vi "Hardware-EPTx-Host.vi"() -> ()   [LabVIEW 2016]
uses:
  <vilib>/Powertrain Controls/Device Drivers/DCM/Rev0/FPGA/Digital Channel.ctl
  <vilib>/Powertrain Controls/Device Drivers/DCM/Rev0/FPGA/DCM - FPGA.lvlib
panel:
  in  "_EPTx Config List":i32(listbox) caption="Deployed EPTx Configurations"
  in  "_Refresh  EPTx Config":bool
  in  "_Open EPTx DB Editor":bool
  out "LoadingSettings":bool
  in  "LoadSettings":bool
  in  "_EPTx Signal Select":T2 caption="EPTx Signal Select"
  in  "HistoryCAD":u8=255
  in  "_Hidden":enum32{"Invisible"}(tab)
  in  "Aux4Select":u8
  in  "Aux3Select":u8
  in  "Aux2Select":u8
  in  "Aux1Select":u8
  in  "PrimarySelect":u8
  out "MaxCAD":sgl
  in  "SimSpeed":sgl
  in  "SimEnable":bool
  in  "SyncEnable":bool
  in  "ClearErrors":bool
  in  "Aux4Filter":sgl format="%#_6p"
  in  "Aux3Filter":sgl format="%#_6p"
  in  "Aux2Filter":sgl format="%#_6p"
  in  "Aux1Filter":sgl format="%#_6p"
  in  "PrimaryFilter":sgl format="%#_6p"
  out "RcvgPrimary":bool
  out "AuxWarning":bool
  out "WatchdogError":bool
  out "Config":bool
  out "PatternError":bool
  out "RatioError":bool
  out "Overflow":bool
  out "Stall":bool
  out "CurrentCAD":sgl
  out "Speed":sgl
  out "Sync":bool
  in  "EPTxSettingsFilename":string="c:\\ni-rt\\LabVIEW Data\\60-2.EPTx"
  out "SYS|Exec|IP_Address":string="10.15.1.12"
  in  "SYS|Exec|Password":string caption="Password"
  in  "SYS|Exec|Username":string="admin" caption="Username"
  in  "_EPTxState":T3 caption="EPTxState"
  out "_EPTx Data":T4 caption="EPTx Data"
  in  "_EPTxFilters":T5 caption="EPTxFilters" {"Aux 4 [s]" format="%#_6p"; "Aux 3 [s]" format="%#_6p"; "Aux 2 [s]" format="%#_6p"; "Aux 1 [s]" format="%#_6p"; "Primary [s]" format="%#_6p"}
  in  "StallSpeed":sgl=500.0
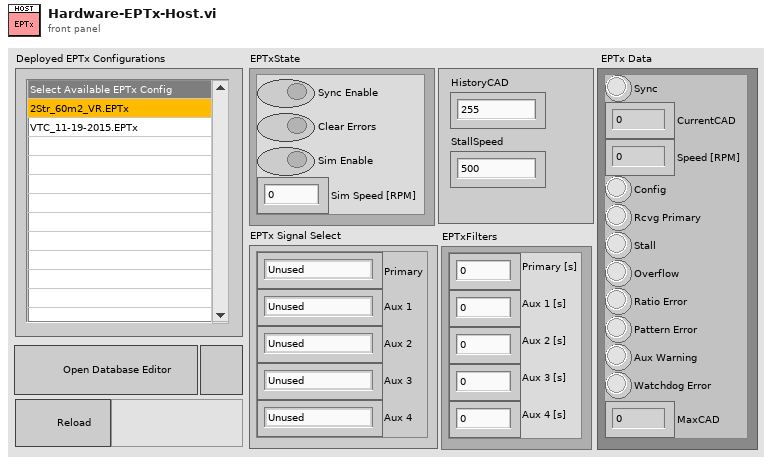
[diagram p1: front panel]
types:
  T1 = typedef "DCM - FPGA.lvlib/Digital Channel.ctl" = enum8{"Unused", "User OS", "Diff IO 1", "Diff IO 2", "Diff IO 3", "Diff IO 4", "Diff IO 5", "Diff IO 6", "Diff IO 7", "Diff IO 8", "Aux 1", "Aux 2", "Aux 3", "Aux 4", "Aux 5", "Aux 6", "Aux 7", "Aux 8", "Aux 9", "Aux 10", "Aux 11", "Aux 12", "Aux 13", "Aux 14", "Aux 15", "Aux 16"}
  T2 = cluster{"Primary":T1, "Aux 1":T1, "Aux 2":T1, "Aux 3":T1, "Aux 4":T1}
  T3 = cluster{"Sync Enable":bool, "Clear Errors":bool, "Sim Enable":bool, "Sim Speed [RPM]":sgl}
  T4 = cluster{"Sync":bool, "CurrentCAD":sgl, "Speed [RPM]":sgl, "Config":bool, "Rcvg Primary":bool, "Stall":bool, "Overflow":bool, "Ratio Error":bool, "Pattern Error":bool, "Aux Warning":bool, "Watchdog Error":bool, "MaxCAD":sgl}
  T5 = cluster{"Primary [s]":sgl, "Aux 1 [s]":sgl, "Aux 2 [s]":sgl, "Aux 3 [s]":sgl, "Aux 4 [s]":sgl}
  T6 = cluster{"PrimarySelect":u8, "Aux1Select":u8, "Aux2Select":u8, "Aux3Select":u8, "Aux4Select":u8}
  T7 = cluster{"PrimaryFilter":sgl, "Aux1Filter":sgl, "Aux2Filter":sgl, "Aux3Filter":sgl, "Aux4Filter":sgl}
  T8 = cluster{"Sync":bool, "CurrentCAD":sgl, "Speed":sgl, "Config":bool, "RcvgPrimary":bool, "Stall":bool, "Overflow":bool, "PatternError":bool, "RatioError":bool, "AuxWarning":bool, "WatchdogError":bool, "MaxCAD":sgl}
  T9 = cluster{"SyncEnable":bool, "ClearErrors":bool, "SimEnable":bool, "SimSpeed":sgl}
  T10 = typedef "LVMinMaxIncTypeDef.ctl" = cluster{"Minimum":dbl, "Maximum":dbl, "Increment":dbl}
  T11 = typedef "LVOutOfRangeActionTypeDef.ctl" = cluster{"OutOfRngActMin":u8, "OutOfRngActMax":u8, "OutOfRngActInc":u8}
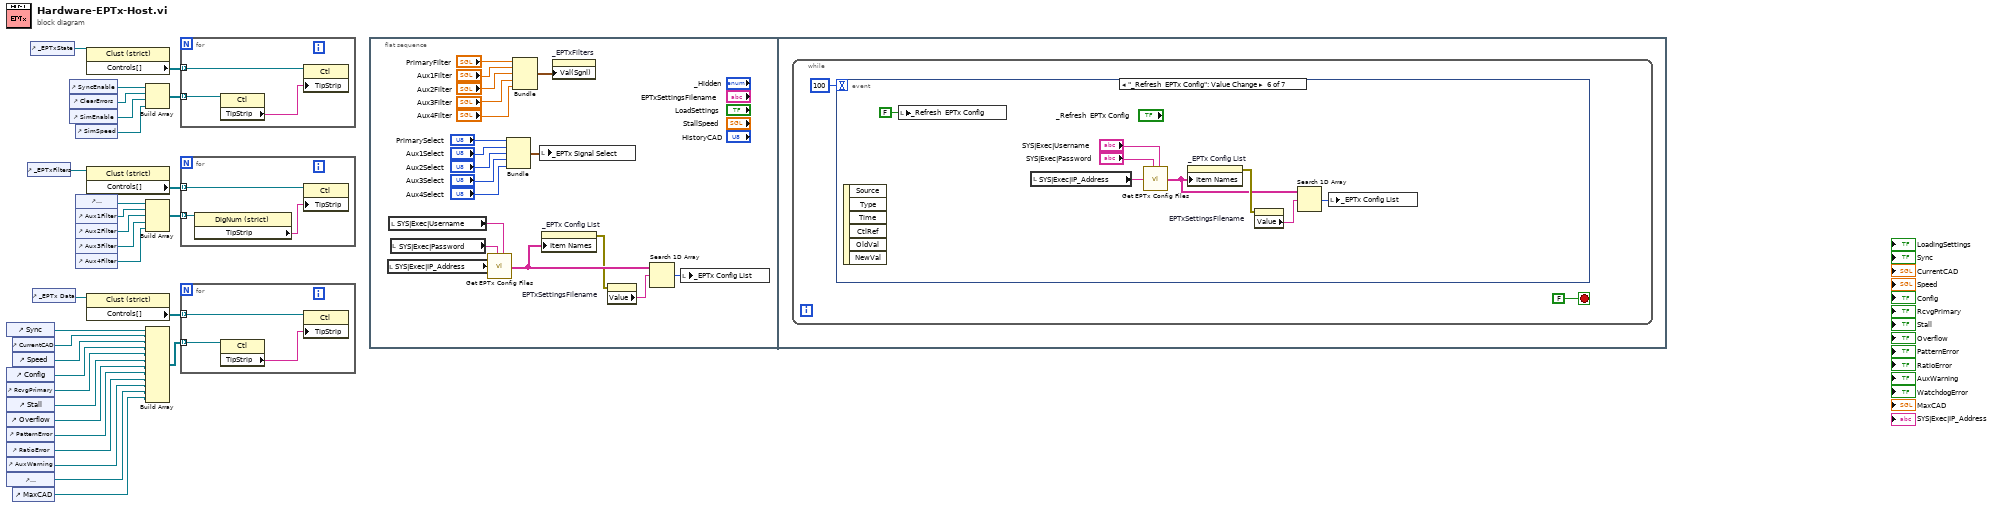
[diagram p0: block diagram]
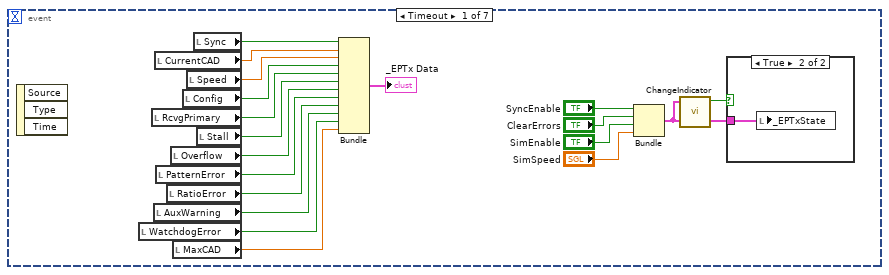
[diagram p2: hidden frame]
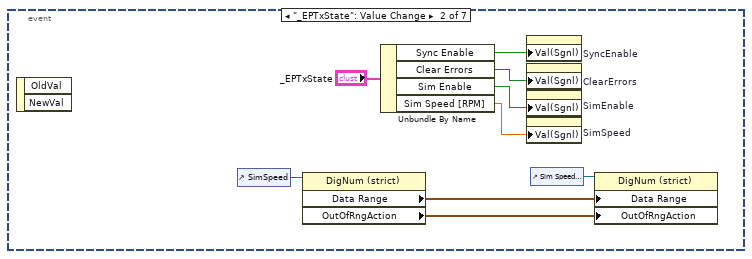
[diagram p4: hidden frame]
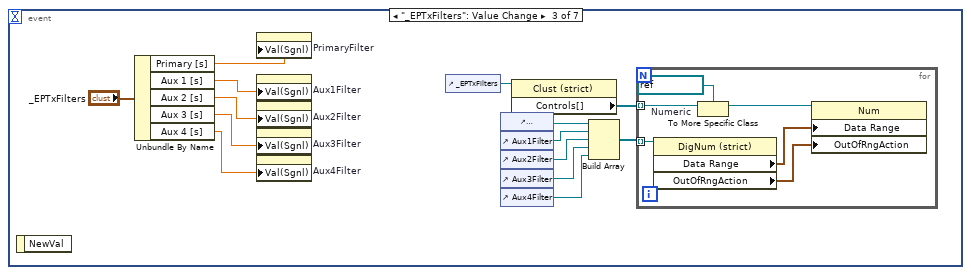
[diagram p5: hidden frame]
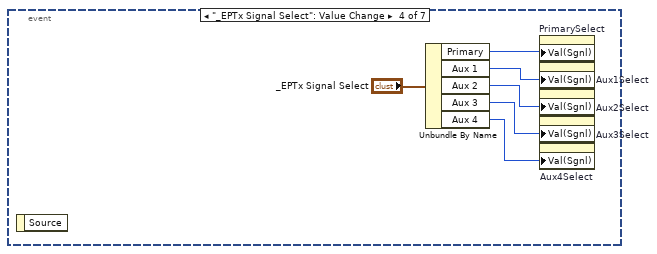
[diagram p6: hidden frame]
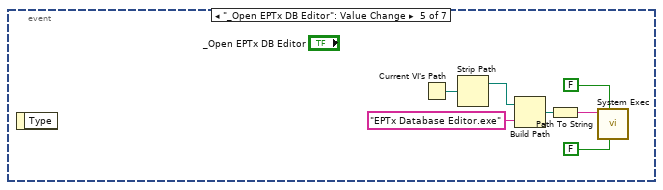
[diagram p7: hidden frame]
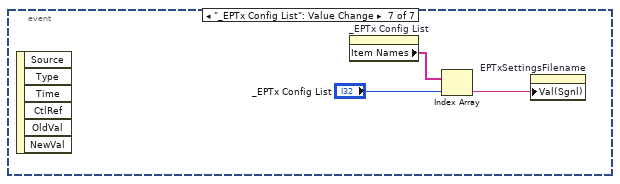
[diagram p8: hidden frame]
diagram:
  n1 = control-ref of="Sync"() -> (w12:refnum<vi>)
  n2 = control-ref of="Config"() -> (w9:refnum<vi>)
  n3 = control-ref of="RcvgPrimary"() -> (w8:refnum<vi>)
  n4 = control-ref of="Stall"() -> (w7:refnum<vi>)
  n5 = control-ref of="Overflow"() -> (w6:refnum<vi>)
  n6 = control-ref of="PatternError"() -> (w5:refnum<vi>)
  n7 = control-ref of="RatioError"() -> (w4:refnum<vi>)
  n8 = control-ref of="AuxWarning"() -> (w3:refnum<vi>)
  n9 = control-ref of="WatchdogError"() -> (w2:refnum<vi>)
  n10 = control-ref of="CurrentCAD"() -> (w11:refnum<vi>)
  n11 = control-ref of="Speed"() -> (w10:refnum<vi>)
  n12 = control-ref of="MaxCAD"() -> (w1:refnum<vi>)
  n13 = control-ref of="_EPTxFilters"() -> (w21:refnum<vi>)
  n14 = control-ref of="_EPTxState"() -> (w28:refnum<vi>)
  n15 = control-ref of="_EPTx Data"() -> (w13:refnum<vi>)
  n16 = control-ref of="SyncEnable"() -> (w27:refnum<vi>)
  n17 = control-ref of="ClearErrors"() -> (w26:refnum<vi>)
  n18 = control-ref of="SimEnable"() -> (w25:refnum<vi>)
  n19 = control-ref of="SimSpeed"() -> (w24:refnum<vi>)
  n20 = control-ref of="PrimaryFilter"() -> (w20:refnum<vi>)
  n21 = control-ref of="Aux1Filter"() -> (w19:refnum<vi>)
  n22 = control-ref of="Aux2Filter"() -> (w18:refnum<vi>)
  n23 = control-ref of="Aux3Filter"() -> (w17:refnum<vi>)
  n24 = control-ref of="Aux4Filter"() -> (w16:refnum<vi>)
  n25 = property on="Property Node" class="Clust (strict)"(reference=w28) -> ("Controls[]"=w30:refnum<vi>[])  [unwired: 1 in, 2 out]
  n26 = property on="Property Node" class="Clust (strict)"(reference=w21) -> ("Controls[]"=w22:refnum<vi>[])  [unwired: 1 in, 2 out]
  n27 = property on="Property Node" class="Clust (strict)"(reference=w13) -> ("Controls[]"=w15:refnum<vi>[])  [unwired: 1 in, 2 out]
  n28 = Build Array(w27, w26, w25, w24) -> (w29:refnum<vi>[])
  n29 = Build Array(w20, w19, w18, w17, w16) -> (w23:refnum<vi>[])
  n30 = Build Array(w12, w11, w10, w9, w8, w7, w6, w5, w4, w3, w2, w1) -> (w14:refnum<vi>[])
  n31 = for {
    tunnel: w30 -> [w33] mode=indexing
    tunnel: w29 -> [w31] mode=indexing
    n32 = property on="Property Node" class="Ctl"(reference=w31) -> ("TipStrip"=w32:string)  [unwired: 1 in, 2 out]
    n33 = property on="Property Node" class="Ctl"(reference=w33, "TipStrip"=w32) -> ()  [unwired: 1 in, 2 out]
  }
  n34 = for {
    tunnel: w22 -> [w36] mode=indexing
    tunnel: w23 -> [w34] mode=indexing
    n35 = property on="Property Node" class="DigNum (strict)"(reference=w34) -> ("TipStrip"=w35:string)  [unwired: 1 in, 2 out]
    n36 = property on="Property Node" class="Ctl"(reference=w36, "TipStrip"=w35) -> ()  [unwired: 1 in, 2 out]
  }
  n37 = for {
    tunnel: w15 -> [w39] mode=indexing
    tunnel: w14 -> [w37] mode=indexing
    n38 = property on="Property Node" class="Ctl"(reference=w37) -> ("TipStrip"=w38:string)  [unwired: 1 in, 2 out]
    n39 = property on="Property Node" class="Ctl"(reference=w39, "TipStrip"=w38) -> ()  [unwired: 1 in, 2 out]
  }
  n40 = flat-sequence {
    frame #0 {
      n41 = local read "SYS|Exec|IP_Address"() -> (w58:string)
      n42 = local read "SYS|Exec|Username"() -> (w56:string)
      n43 = local read "SYS|Exec|Password"() -> (w57:string)
      n44 = call "Get EPTx Config Files.vi"("password"=w57, "IP_Address"=w58, "username"=w56) -> ("EPTx Files"=w53:string[])  [unwired: 6 in]
      n45 = Bundle("PrimarySelect"="PrimarySelect", "Aux1Select"="Aux1Select", "Aux2Select"="Aux2Select", "Aux3Select"="Aux3Select", "Aux4Select"="Aux4Select") -> (w51:T6)  [unwired: 1 in]
      n46 = Bundle("PrimaryFilter"="PrimaryFilter", "Aux1Filter"="Aux1Filter", "Aux2Filter"="Aux2Filter", "Aux3Filter"="Aux3Filter", "Aux4Filter"="Aux4Filter") -> (w45:T7)  [unwired: 1 in]
      n47 = local write "_EPTx Signal Select"(w51) -> ()
      n48 = property on="_EPTx Config List" class="LstBox (strict)"("Item Names"=w53) -> (error out=w52:errorcluster)  [unwired: 2 in, 1 out]
      n49 = property on="_EPTxFilters" class="Clust (strict)"("Val(Sgnl)"=w45) -> ()  [unwired: 2 in, 2 out]
      n50 = property on="EPTxSettingsFilename" class="Str"(error in=w52) -> ("Value"=w55:string)  [unwired: 1 in, 2 out]
      n51 = Search 1D Array(1D array=w53, element=w55) -> (index of element=w54:i32)  [unwired: 1 in]
      n52 = local write "_EPTx Config List"(w54) -> ()
    }
    frame #1 {
      n53 = while {
        stop <- FALSE stop-if-true
        n54 = event shown="[5] \"_Refresh  EPTx Config\": Value Change" {
          selector: _ -> [_ _ _ _ _ _ _]
          dyn-events: _ -> [_ _ _ _ _ _ _]
          timeout: 100 -> [_ _ _ _ _ _ _]
          event Timeout {
            n55 = event-data() -> ()  [unwired: 1 in, 3 out]
            n56 = local read "WatchdogError"() -> (w79:bool)
            n57 = local read "RcvgPrimary"() -> (w73:bool)
            n58 = local read "AuxWarning"() -> (w78:bool)
            n59 = local read "CurrentCAD"() -> (w70:sgl)
            n60 = local read "PatternError"() -> (w76:bool)
            n61 = local read "RatioError"() -> (w77:bool)
            n62 = local read "Overflow"() -> (w75:bool)
            n63 = local read "MaxCAD"() -> (w68:sgl)
            n64 = local read "Config"() -> (w72:bool)
            n65 = local read "Speed"() -> (w71:sgl)
            n66 = local read "Sync"() -> (w69:bool)
            n67 = local read "Stall"() -> (w74:bool)
            n68 = Bundle("Sync"=w69, "CurrentCAD"=w70, "Speed"=w71, "Config"=w72, "RcvgPrimary"=w73, "Stall"=w74, "Overflow"=w75, "PatternError"=w76, "RatioError"=w77, "AuxWarning"=w78, "WatchdogError"=w79, "MaxCAD"=w68) -> (→"_EPTx Data":T8)  [unwired: 1 in]
            n69 = Bundle("SyncEnable"="SyncEnable", "ClearErrors"="ClearErrors", "SimEnable"="SimEnable", "SimSpeed"="SimSpeed") -> (w62:T9)  [unwired: 1 in]
            n70 = call "ChangeIndicator.vi"("Input"=w62) -> ("Change"=w61:bool)  [unwired: 9 in]
            n71 = case shown="True" w61 {
              tunnel: w62 -> [_ w80]
              frame False {
              }
              frame True {
                n72 = local write "_EPTxState"(w80) -> ()
              }
            }
          }
          event "_EPTxState": Value Change {
            n73 = event-data() -> ()  [unwired: 1 in, 2 out]
            n74 = control-ref of="SimSpeed"() -> (w84:refnum<vi>)
            n75 = property on="Property Node" class="DigNum (strict)"(reference=w84) -> ("Data Range"=w82:T10, "OutOfRngAction"=w81:T11)  [unwired: 1 in, 2 out]
            n76 = Unbundle By Name("_EPTxState") -> ("Sync Enable"=w86:bool, "Clear Errors"=w87:bool, "Sim Enable"=w88:bool, "Sim Speed [RPM]"=w89:sgl)
            n77 = property on="SyncEnable" class="Bool (strict)"("Val(Sgnl)"=w86) -> ()  [unwired: 2 in, 2 out]
            n78 = property on="ClearErrors" class="Bool (strict)"("Val(Sgnl)"=w87) -> ()  [unwired: 2 in, 2 out]
            n79 = property on="SimEnable" class="Bool (strict)"("Val(Sgnl)"=w88) -> ()  [unwired: 2 in, 2 out]
            n80 = property on="SimSpeed" class="DigNum (strict)"("Val(Sgnl)"=w89) -> ()  [unwired: 2 in, 2 out]
            n81 = control-ref of="Sim Speed [RPM]"() -> (w83:refnum<vi>)
            n82 = property on="Property Node" class="DigNum (strict)"(reference=w83, "Data Range"=w82, "OutOfRngAction"=w81) -> ()  [unwired: 1 in, 2 out]
          }
          event "_EPTxFilters": Value Change {
            n83 = event-data() -> ()  [unwired: 1 in, 1 out]
            n84 = Unbundle By Name("_EPTxFilters") -> ("Primary [s]"=w99:sgl, "Aux 1 [s]"=w100:sgl, "Aux 2 [s]"=w101:sgl, "Aux 3 [s]"=w102:sgl, "Aux 4 [s]"=w103:sgl)
            n85 = property on="PrimaryFilter" class="DigNum (strict)"("Val(Sgnl)"=w99) -> ()  [unwired: 2 in, 2 out]
            n86 = property on="Aux1Filter" class="DigNum (strict)"("Val(Sgnl)"=w100) -> ()  [unwired: 2 in, 2 out]
            n87 = property on="Aux2Filter" class="DigNum (strict)"("Val(Sgnl)"=w101) -> ()  [unwired: 2 in, 2 out]
            n88 = property on="Aux3Filter" class="DigNum (strict)"("Val(Sgnl)"=w102) -> ()  [unwired: 2 in, 2 out]
            n89 = property on="Aux4Filter" class="DigNum (strict)"("Val(Sgnl)"=w103) -> ()  [unwired: 2 in, 2 out]
            n90 = control-ref of="_EPTxFilters"() -> (w90:refnum<vi>)
            n91 = control-ref of="PrimaryFilter"() -> (w92:refnum<vi>)
            n92 = control-ref of="Aux1Filter"() -> (w93:refnum<vi>)
            n93 = control-ref of="Aux2Filter"() -> (w94:refnum<vi>)
            n94 = control-ref of="Aux3Filter"() -> (w95:refnum<vi>)
            n95 = control-ref of="Aux4Filter"() -> (w96:refnum<vi>)
            n96 = property on="Property Node" class="Clust (strict)"(reference=w90) -> ("Controls[]"=w97:refnum<vi>[])  [unwired: 1 in, 2 out]
            n97 = Build Array(w92, w93, w94, w95, w96) -> (w91:refnum<vi>[])
            n98 = for {
              tunnel: w97 -> [w109] mode=indexing
              tunnel: w91 -> [w108] mode=indexing
              w106 = refnum<vi> refnum  # Numeric
              n99 = property on="Property Node" class="DigNum (strict)"(reference=w108) -> ("Data Range"=w105:T10, "OutOfRngAction"=w104:T11)  [unwired: 1 in, 2 out]
              n100 = To More Specific Class(target class=w106, reference=w109) -> (specific class reference=w107:refnum<vi>)  [unwired: 1 in, 1 out]
              n101 = property on="Property Node" class="Num"(reference=w107, "Data Range"=w105, "OutOfRngAction"=w104) -> ()  [unwired: 1 in, 2 out]
            }
          }
          event "_EPTx Signal Select": Value Change {
            n102 = event-data() -> ()  [unwired: 1 in, 1 out]
            n103 = Unbundle By Name("_EPTx Signal Select") -> ("Primary"=w111:T1, "Aux 1"=w112:T1, "Aux 2"=w113:T1, "Aux 3"=w114:T1, "Aux 4"=w115:T1)
            n104 = property on="PrimarySelect" class="DigNum (strict)"("Val(Sgnl)"=w111) -> ()  [unwired: 2 in, 2 out]
            n105 = property on="Aux1Select" class="DigNum (strict)"("Val(Sgnl)"=w112) -> ()  [unwired: 2 in, 2 out]
            n106 = property on="Aux2Select" class="DigNum (strict)"("Val(Sgnl)"=w113) -> ()  [unwired: 2 in, 2 out]
            n107 = property on="Aux3Select" class="DigNum (strict)"("Val(Sgnl)"=w114) -> ()  [unwired: 2 in, 2 out]
            n108 = property on="Aux4Select" class="DigNum (strict)"("Val(Sgnl)"=w115) -> ()  [unwired: 2 in, 2 out]
          }
          event "_Open EPTx DB Editor": Value Change {
            n109 = event-data() -> ()  [unwired: 1 in, 1 out]
            n110 = Current VI's Path() -> (path=w117:path)
            n111 = Strip Path(path=w117) -> (stripped path=w116:path)  [unwired: 1 out]
            n112 = Build Path(base path=w116, name or relative path="EPTx Database Editor.exe") -> (appended path=w122:path)
            n113 = Path To String(path=w122) -> (string=w119:string)
            n114 = call <vilib>:"System Exec.vi"("run minimized? (F)"=FALSE, "wait until completion? (T)"=FALSE, "command line"=w119) -> ()  [unwired: 5 in, 4 out]
          }
          event "_Refresh  EPTx Config": Value Change {
            n115 = event-data() -> ()  [unwired: 1 in, 6 out]
            n116 = local write "_Refresh  EPTx Config"(FALSE ("_Refresh  EPTx Config")) -> ()
            n117 = local read "SYS|Exec|IP_Address"() -> (w129:string)
            n118 = call "Get EPTx Config Files.vi"("password"="SYS|Exec|Password", "IP_Address"=w129, "username"="SYS|Exec|Username") -> ("EPTx Files"=w123:string[])  [unwired: 6 in]
            n119 = property on="_EPTx Config List" class="LstBox (strict)"("Item Names"=w123) -> (error out=w124:errorcluster)  [unwired: 2 in, 1 out]
            n120 = property on="EPTxSettingsFilename" class="Str"(error in=w124) -> ("Value"=w125:string)  [unwired: 1 in, 2 out]
            n121 = Search 1D Array(1D array=w123, element=w125) -> (index of element=w126:i32)  [unwired: 1 in]
            n122 = local write "_EPTx Config List"(w126) -> ()
          }
          event "_EPTx Config List": Value Change {
            n123 = event-data() -> ()  [unwired: 1 in, 6 out]
            n124 = property on="_EPTx Config List" class="LstBox (strict)"() -> ("Item Names"=w131:string[])  [unwired: 2 in, 2 out]
            n125 = Index Array(array=w131, index="_EPTx Config List") -> (element=w132:string)
            n126 = property on="EPTxSettingsFilename" class="Str"("Val(Sgnl)"=w132) -> ()  [unwired: 2 in, 2 out]
          }
        }
      }
    }
  }
